vi "emi_Parse String Number List.vi"(7 "Number List(\"0\")":string="0", 11 "error in (no error)":errorcluster) -> (8 "Number Array":i32[](array[numeric]), 15 "error out":errorcluster)   [LabVIEW 2010]
doc: "Accepts a string of the form: \"1,4,6,8-12,56,43,6,122-126\". Truns it in to an array of I32;\n1;4;6;8;9;10;11;12;56;43;6;122;123;124;125;126.\n\nThere is no limit to number of \"numbers\" but be aware of increased processing times at larger sets(1000+). White spaces are all removed befor processing.\n\nComma delimiters excepted: \",\" \";\" \":\" \".\"\nSpan delimeters excepted: \"-\" \"_\"\n\n\nOn Error: No Action"
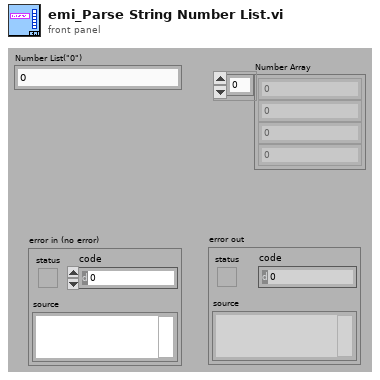
[diagram p1: front panel]
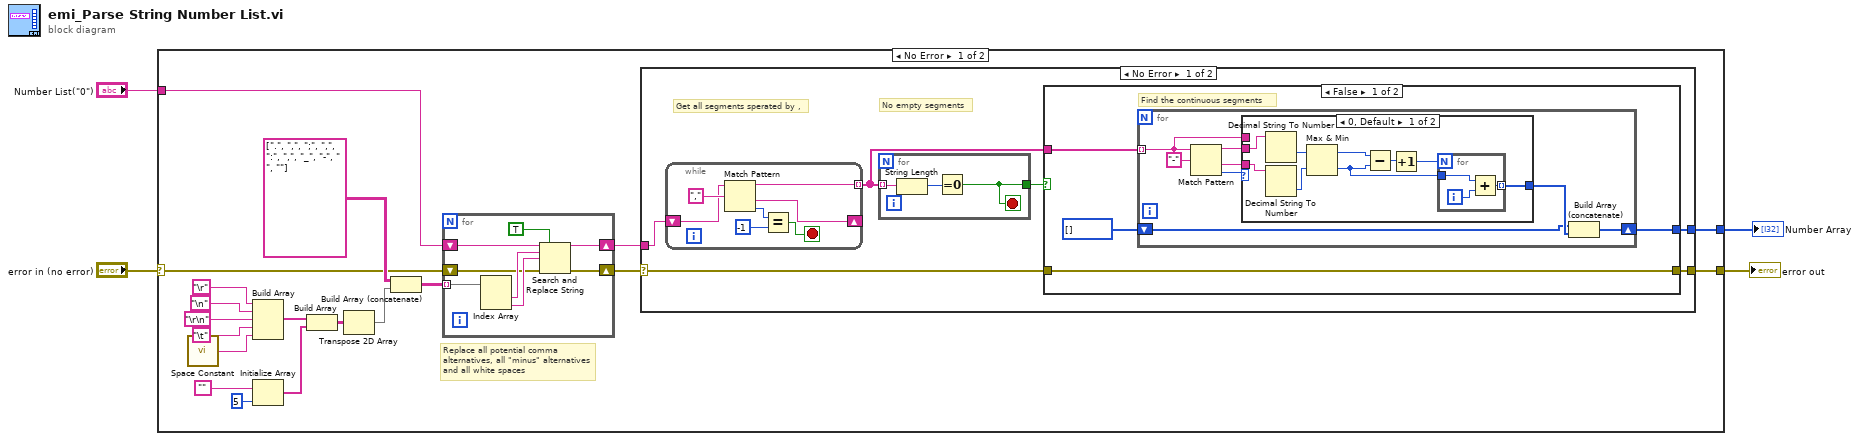
[diagram p0: block diagram]
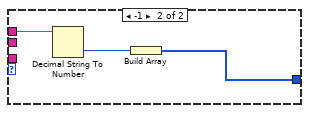
[diagram p2: hidden frame]
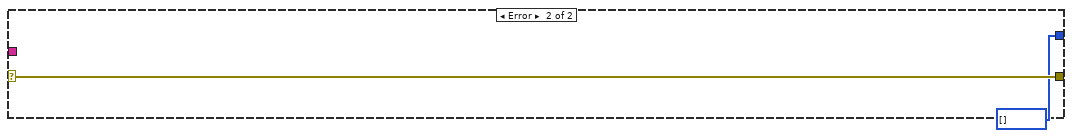
[diagram p4: hidden frame]
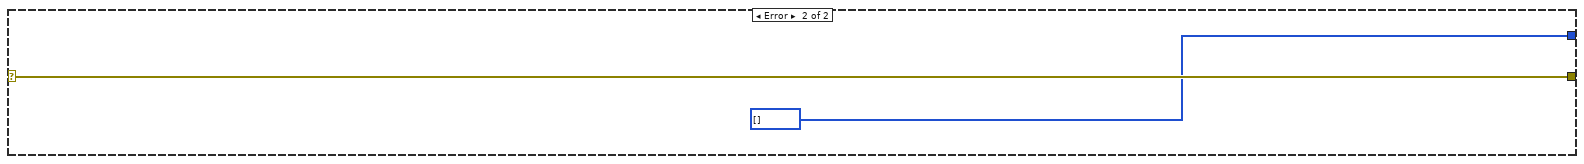
[diagram p5: hidden frame]
diagram:
  n1 = case shown="No Error" "error in (no error)" {
    selector: "error in (no error)" -> [w7 w80]
    tunnel: "Number List(\"0\")" -> [w11 _]
    tunnel: [w8 i32[] [] ("appended array")] -> w3
    tunnel: [w5 w80] -> w1
    frame No Error {
      # "Replace all potential comma \nalternatives, all \"minus\" alternatives\nand all white spaces"
      n2 = call <vilib>:"Space Constant.vi"() -> ("String"=w19:string)
      n3 = Build Array("\r", "\n", "\r\n", "\t", w19) -> (w18:string[])
      n4 = Initialize Array("", 5 ("dimension size")) -> (w15:string[])
      n5 = Build Array(w18, w15) -> (w14:string[][])
      n6 = Transpose 2D Array(2D array=w14) -> (transposed array=w12:string[][])
      n7 = Build Array (concatenate)(string[][] [[".", ","], [";", ","], [":", ","], ["_", "-"], [" ", ""]], w12) -> (w10:string[][])
      n8 = for {
        tunnel: w10 -> [w77] mode=indexing
        shift-right: [w74] -> w9
        shift-left: w11 -> [w78]
        shift-right: [w71] -> w6
        shift-left: w7 -> [w72]
        n9 = Index Array(array=w77) -> (element #1=w76:string, element #2=w75:string)  [unwired: 2 in]
        n10 = Search and Replace String(replace all?=TRUE ("replace all? (F)"), input string=w78, search string=w76, replace string=w75, error in=w72) -> (result string=w74:string, error out=w71:errorcluster)  [unwired: 3 in, 2 out]
      }
      n11 = case shown="No Error" w6 {
        selector: w6 -> [w25 w70]
        tunnel: w9 -> [w29 _]
        tunnel: [w28 i32[] [] ("appended array")] -> w8
        tunnel: [w24 w70] -> w5
        frame No Error {
          # "No empty segments"
          # "Get all segments sperated by ,"
          n12 = while {
            shift-right: [w66] -> _
            shift-left: w29 -> [w67]
            tunnel: [w65] -> w27 mode=indexing
            stop <- w64 stop-if-true
            n13 = Match Pattern(string=w67, regular expression="," ("search string/char (-)")) -> (before substring=w65:string, after substring=w66:string, offset past match=w63:i32)  [unwired: 1 in, 1 out]
            n14 = Equal?(x=w63, y=-1) -> (x = y?=w64:bool)
          }
          n15 = for {
            tunnel: w27 -> [w32] mode=indexing
            tunnel: [w30] -> w26
            stop <- w30 stop-if-true
            n16 = String Length(string=w32) -> (length=w31:i32)
            n17 = Equal To 0?(x=w31) -> (x = 0?=w30:bool)
          }
          n18 = case shown="False" w26 {
            tunnel: w27 -> [w36 _]
            tunnel: [w34 i32[] [] ("appended array")] -> w28
            tunnel: w25 -> [w33 w60]
            tunnel: [w33 w60] -> w24
            frame False {
              # "Find the continuous segments"
              n19 = for {
                tunnel: w36 -> [w42] mode=indexing
                shift-right: [w37] -> w34
                shift-left: i32[] [] ("appended array") -> [w38]
                n20 = Match Pattern(string=w42, regular expression="-") -> (before substring=w41:string, after substring=w40:string, offset past match=w43:i32)  [unwired: 1 in, 1 out]
                n21 = case shown="0, Default" w43 {
                  tunnel: w42 -> [_ w59]
                  tunnel: w41 -> [w53 _]
                  tunnel: w40 -> [w52 _]
                  tunnel: [w46 w57] -> w39
                  frame 0, Default {
                    n22 = Decimal String To Number(string=w53) -> (number=w51:i32)  [unwired: 2 in, 1 out]
                    n23 = Decimal String To Number(string=w52) -> (number=w50:i32)  [unwired: 2 in, 1 out]
                    n24 = Max & Min(x=w51, y=w50) -> (max(x,y)=w49:i32, min(x,y)=w47:i32)
                    n25 = Subtract(x=w49, y=w47) -> (x-y=w48:i32)
                    n26 = Increment(x=w48) -> (x+1=w45:i32)
                    n27 = for {
                      N: w45 -> [_]
                      tunnel: w47 -> [w56]
                      tunnel: [w54] -> w46 mode=indexing
                      i -> [w55]
                      n28 = Add(x=w56, y=w55) -> (x+y=w54:i32)
                    }
                  }
                  frame -1 {
                    n29 = Decimal String To Number(string=w59) -> (number=w58:i32)  [unwired: 2 in, 1 out]
                    n30 = Build Array(w58) -> (w57:i32[])
                  }
                }
                n31 = Build Array (concatenate)(w38, w39) -> (w37:i32[])
              }
            }
            frame True {
            }
          }
        }
        frame Error {
        }
      }
    }
    frame Error {
    }
  }
  "Number Array" <- w3
  "error out" <- w1
